vi "DPT TC Panel Parser.vi"(9 "Index start":i32, 10 "Panel Num":string, 11 "TC Panel 1":T2[][](array[typedef])=[[{"Label"="RDB F", "Record"=TRUE, "Index"=0, "Channel"=""}, {"Label"="Room Ambient(F)", "Record"=TRUE, "Index"=0, "Channel"=""}, {"Label"="Tscale", "Record"=TRUE, "Index"=0, "Channel"=""}, {"Label"="", "Record"=FALSE, "Index"=0, "Channel"=""}, {"Label"="", "Record"=FALSE, "Index"=0, "Channel"=""}, {"Label"="", "Record"=FALSE, "Index"=0, "Channel"=""}], [{"Label"="", "Record"=FALSE, "Index"=0, "Channel"=""}, {"Label"="", "Record"=FALSE, "Index"=0, "Channel"=""}, {"Label"="", "Record"=FALSE, "Index"=0, "Channel"=""}, {"Label"="", "Record"=FALSE, "Index"=0, "Channel"=""}, {"Label"="", "Record"=FALSE, "Index"=0, "Channel"=""}, {"Label"="", "Record"=FALSE, "Index"=0, "Channel"=""}], [{"Label"="", "Record"=FALSE, "Index"=0, "Channel"=""}, {"Label"="", "Record"=FALSE, "Index"=0, "Channel"=""}, {"Label"="", "Record"=FALSE, "Index"=0, "Channel"=""}, {"Label"="", "Record"=FALSE, "Index"=0, "Channel"=""}, {"Label"="", "Record"=FALSE, "Index"=0, "Channel"=""}, {"Label"="", "Record"=FALSE, "Index"=0, "Channel"=""}]]) -> (0 "Indexes Used":i32[](array[numeric]), 1 "Channel Array":string[](array[string]), 2 "Label Array":T1[](array[typedef]))   [LabVIEW 2016]
doc: "Analyzes panel control element's data and separates it into 3 categories: Panel location, Label name, Channel number"
uses:
  Type Definitions/DPT Channel Label.ctl
  Utility/Custom Pallet Controls/Custom Pallet String.ctl
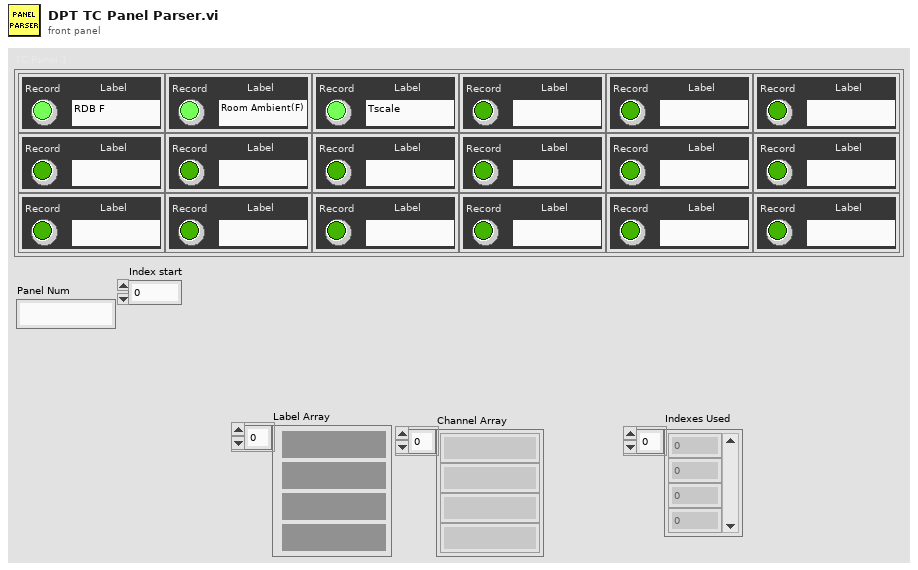
[diagram p1: front panel]
types:
  T1 = typedef "Custom Pallet String.ctl" = string
  T2 = typedef "DPT Channel Label.ctl" = cluster{"Label":T1, "Record":bool, "Index":u32, "Channel":string}
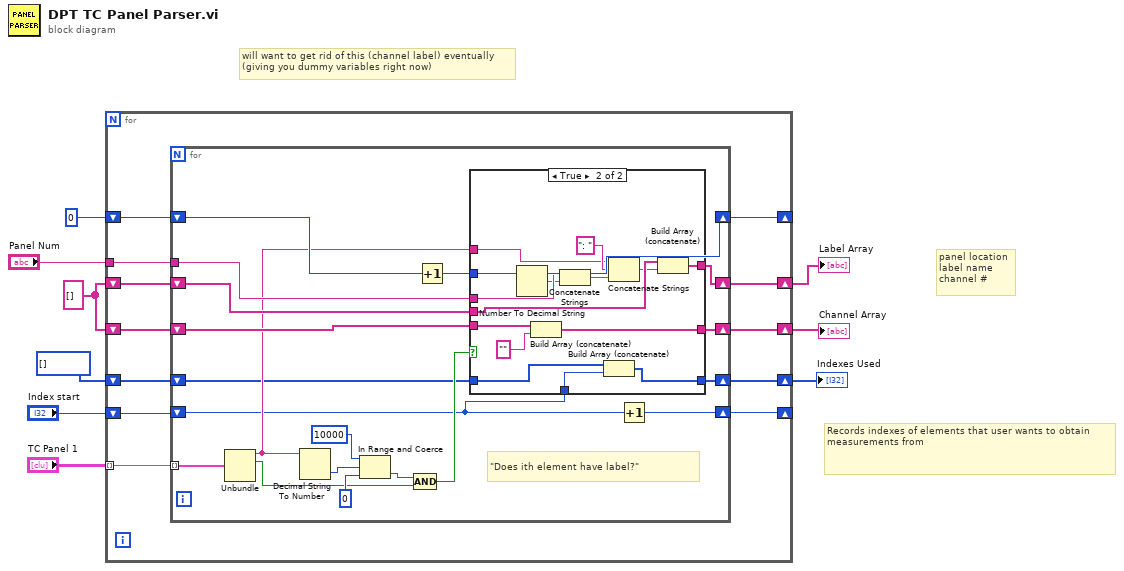
[diagram p0: block diagram]
diagram:
  w2 = string[] []
  # "Records indexes of elements that user wants to obtain measurements from"
  # "panel location\nlabel name\nchannel #"
  # "will want to get rid of this (channel label) eventually\n(giving you dummy variables right now)"
  n1 = for {
    tunnel: "TC Panel 1" -> [w21] mode=indexing
    shift-right: [w20] -> w9
    shift-left: w2 -> [w19]
    shift-right: [w18] -> w8
    shift-left: w2 -> [w17]
    shift-right: [w15] -> _
    shift-left: 0 -> [w16]
    tunnel: "Panel Num" -> [w10]
    shift-right: [w14] -> w5
    shift-left: i32[] [] -> [w13]
    shift-right: [w11] -> _
    shift-left: "Index start" -> [w12]
    n2 = for {
      tunnel: w21 -> [w40] mode=indexing
      shift-right: [w38] -> w20
      shift-left: w19 -> [w36]
      shift-right: [w34] -> w18
      shift-left: w17 -> [w35]
      shift-right: [w37] -> w15
      shift-left: w16 -> [w39]
      tunnel: w10 -> [w33]
      shift-right: [w25] -> w14
      shift-left: w13 -> [w24]
      shift-right: [w22] -> w11
      shift-left: w12 -> [w23]
      # "\"Does ith element have label?\""
      n3 = Unbundle(w40) -> ("Label"=w29:T1, "Record"=w27:bool)  [unwired: 2 out]
      n4 = Decimal String To Number(string=w29) -> (number=w32:i32)  [unwired: 2 in, 1 out]
      n5 = In Range and Coerce(upper limit=10000, x=w32, lower limit=0) -> (In Range?=w30:bool)  [unwired: 1 out]
      n6 = Compound Arithmetic op=AND(w30, w27) -> (w26:bool)
      n7 = Increment(x=w39) -> (x+1=w37:i32)
      n8 = case shown="True" w26 {
        tunnel: [w43 w58] -> w38
        tunnel: w37 -> [_ w57]
        tunnel: w36 -> [w43 w56]
        tunnel: w35 -> [w42 w55]
        tunnel: [w42 w54] -> w34
        tunnel: w33 -> [_ w53]
        tunnel: w29 -> [_ w45]
        tunnel: w23 -> [_ w49]
        tunnel: [w41 w48] -> w25
        tunnel: w24 -> [w41 w50]
        frame False {
        }
        frame True {
          n9 = Number To Decimal String(number=w57) -> (decimal integer string=w52:string)  [unwired: 1 in]
          n10 = Build Array (concatenate)(w55, "") -> (w54:string[])
          n11 = Concatenate Strings(w53, w52) -> (w46:string)
          n12 = Build Array (concatenate)(w50, w49) -> (w48:i32[])
          n13 = Concatenate Strings(w45, ": " ("string"), w46) -> (w44:string)
          n14 = Build Array (concatenate)(w56, w44) -> (w58:string[])
        }
      }
      n15 = Increment(x=w23) -> (x+1=w22:i32)
    }
  }
  "Label Array" <- w9
  "Channel Array" <- w8
  "Indexes Used" <- w5
